vi "LAB_VIWE_USING_OF_MATHAMATICAL_OPERATOR.vi"() -> ()   [LabVIEW 2020]
panel:
  out "DIVISION":dbl
  out "MULTIPLICATION":dbl
  out "SUBSTACTION":dbl
  out "ADDITION":dbl
  in  "NUM 2":dbl
  in  "NUM1":dbl
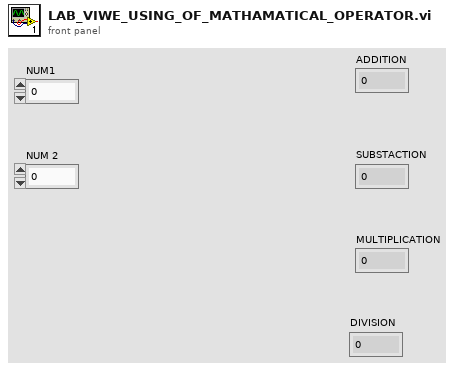
[diagram p1: front panel]
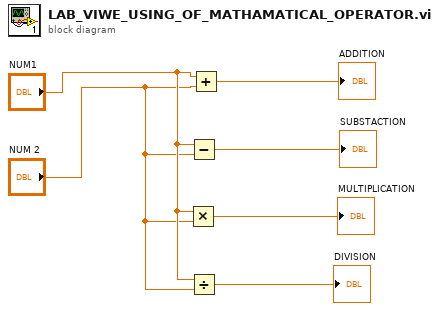
[diagram p0: block diagram]
diagram:
  n1 = Multiply(x="NUM1", y="NUM 2") -> (x*y=→"MULTIPLICATION":dbl)
  n2 = Subtract(x="NUM1", y="NUM 2") -> (x-y=→"SUBSTACTION":dbl)
  n3 = Divide(x="NUM1", y="NUM 2") -> (x/y=→"DIVISION":dbl)
  n4 = Add(x="NUM1", y="NUM 2") -> (x+y=→"ADDITION":dbl)
